vi "cutoff frequency detector.vi"() -> ()   [LabVIEW 2023]
uses:
  ps2000.dll
panel:
  out "Range":dbl
  out "min value":dbl
  out "max value":dbl
  out "Return":string
  in  "error in (no error)":errorcluster
  out "error out":errorcluster
  in  "stop":bool
  out "Waveform Graph":dbl[](graph)
  in  "Trigger Config":T1={"Delay"=0, "Auto_trigger_ms"=0, "Direction"=0, "Source"=5, "Voltage mV"=10} {"Voltage mV" min=0 max=20000 step=50; "Source" items=["Channel A"=0, "Channel B"=1, "Off"=5]; "Direction" items=["Rising", "Falling"]}
  in  "Timebase":cluster{"no_of_samples":i16, "Timebase":i16}
  in  "Apply settings":bool
  in  "Channel A":T2 {"Coupling" items=["DC", "AC"]; "Range" items=["±20 mV"=1, "±50 mV"=2, "±100 mV"=3, "±200 mV"=4, "±500 mV"=5, "±1 V"=6, "±2 V"=7, "±5 V"=8, "±10 V"=9, "±20 V"=10]}
  in  "Channel (1:Channel 1)":u16(ring) items=["", "Channel 1", "Channel 2"]
  in  "DG811 Config":T3
  in  "Waveform Function (0: Sine)":u16(ring) items=["Sine", "Square", "Ramp", "Pulse", "Noise", "DC "]
  in  "Address":refnum<visa-resource-name>
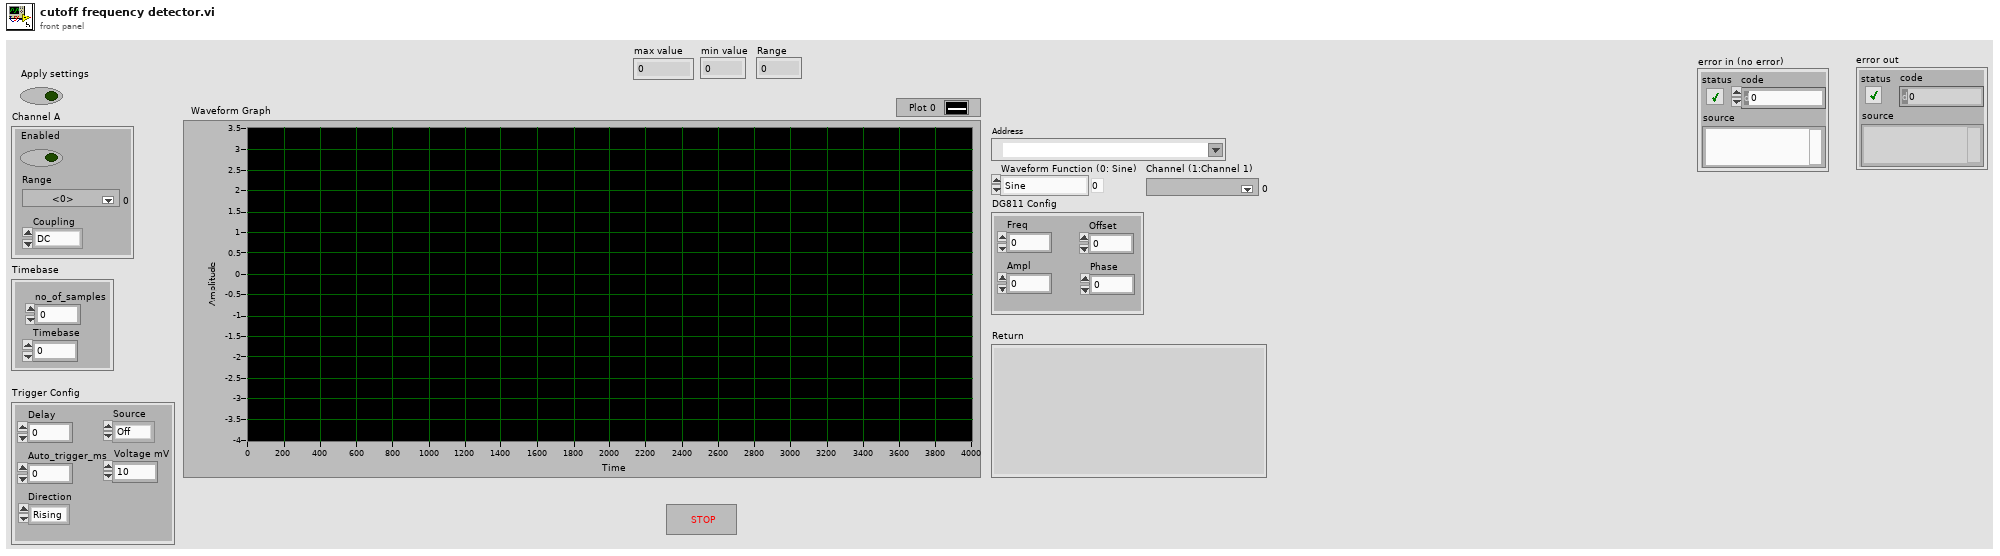
[diagram p1: front panel]
types:
  T1 = cluster{"Delay":i16, "Auto_trigger_ms":i16, "Direction":i16, "Source":i16, "Voltage mV":i16}
  T2 = cluster{"Range":i16, "Enabled":bool, "Coupling":i16}
  T3 = cluster{"Offset ":i8, "Phase ":i8, "Ampl ":i8, "Freq ":i16}
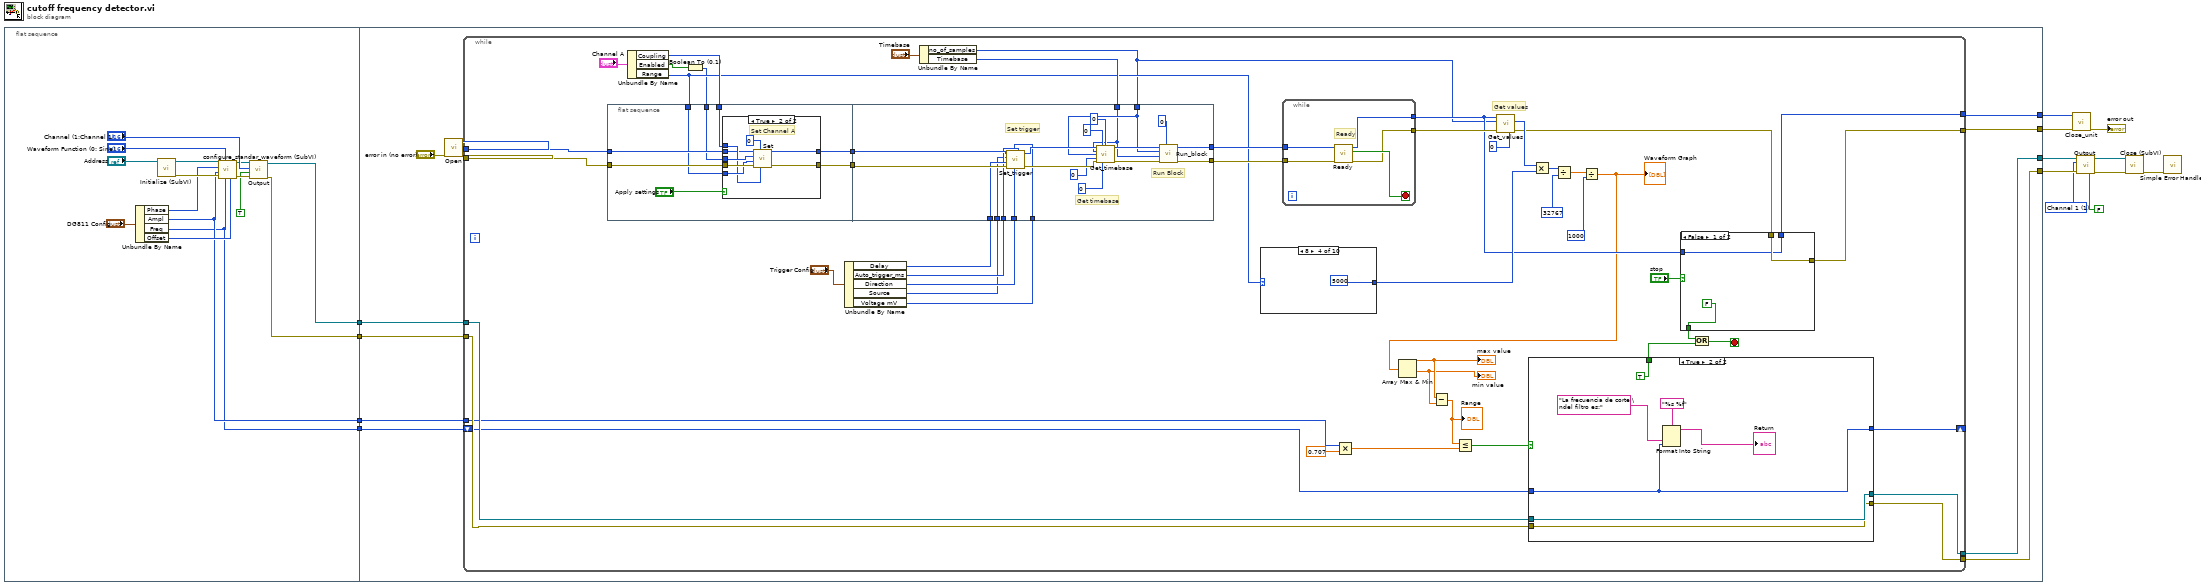
[diagram p0: block diagram]
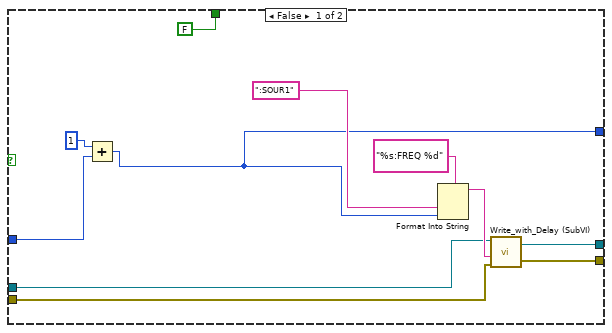
[diagram p2: hidden frame]
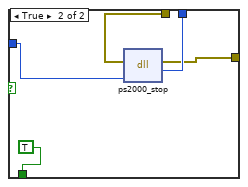
[diagram p3: hidden frame]
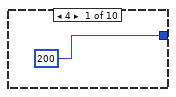
[diagram p5: hidden frame]
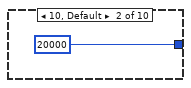
[diagram p6: hidden frame]
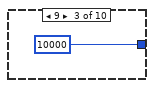
[diagram p7: hidden frame]
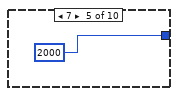
[diagram p8: hidden frame]
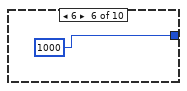
[diagram p9: hidden frame]
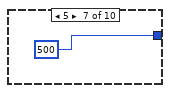
[diagram p10: hidden frame]
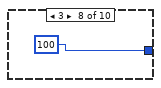
[diagram p11: hidden frame]
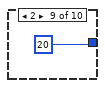
[diagram p12: hidden frame]
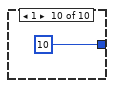
[diagram p13: hidden frame]
diagram:
  w5 = 1 items=["", "Channel 1", "Channel 2"] ("Channel (0: Channel 1)")
  n1 = flat-sequence {
    tunnel: [w22] -> w10
    tunnel: [w21] -> w9
    tunnel: [w16] -> w8
    tunnel: [w15] -> w1
    tunnel: [w37] -> w12
    tunnel: [w36] -> w11
    tunnel: w10 -> [w35]
    tunnel: w9 -> [w34]
    tunnel: [w33] -> w7
    tunnel: [w32] -> w6
    tunnel: w8 -> [w31]
    tunnel: w1 -> [w30]
    frame #0 {
      n2 = Unbundle By Name("DG811 Config") -> ("Phase"=w18:i8, "Ampl"=w16:i8, "Freq"=w15:i16, "Offset"=w17:i8)
      n3 = call "Initialize (SubVI).vi"("VISA Refnum in"="Address") -> ("error out"=w26:errorcluster, "VISA Refnum out"=w25:refnum<visa-resource-name>)  [unwired: 9 in]
      n4 = call "configure_standar_waveform (SubVI).vi"("DC Offset (0 V)"=w17, "Frequency (1000 Hz)"=w15, "Waveform Function (0: Sine) in"="Waveform Function (0: Sine)", "error in (no error)"=w26, "Amplitude (5.0 Vpp)"=w16, "Phase"=w18, "VISA Refnum in"=w25) -> ("error out"=w27:errorcluster, "VISA Refnum out"=w28:refnum<visa-resource-name>)  [unwired: 3 in]
      n5 = call "Output.vi"("error in (no error)"=w27, "Enable Output (T: Enable)"=TRUE, "Channel (0: Channel 1)"="Channel (1:Channel 1)", "VISA Refnum in"=w28) -> ("error out"=w21:errorcluster, "VISA Refnum out"=w22:refnum<visa-resource-name>)  [unwired: 6 in]
    }
    frame #1 {
      n6 = call "Open.vi"("error in (no error)"="error in (no error)") -> ("error out"=w39:errorcluster, "return type"=w38:i16)  [unwired: 9 in]
      n7 = while {
        tunnel: [w78] -> w36
        tunnel: w39 -> [w81]
        tunnel: w38 -> [w82]
        tunnel: [w77] -> w37
        tunnel: w35 -> [w59]
        tunnel: w34 -> [w58]
        tunnel: [w60] -> w33
        tunnel: [w61] -> w32
        tunnel: w31 -> [w46]
        shift-right: [w57] -> _
        shift-left: w30 -> [w56]
        stop <- w54 stop-if-true
        # "Get values"
        n8 = flat-sequence {
          tunnel: w81 -> [w128]
          tunnel: [w127] -> w90
          tunnel: [w126] -> w89
          tunnel: w82 -> [w125]
          tunnel: w73 -> [w124]
          tunnel: w72 -> [w123]
          tunnel: w70 -> [w122]
          tunnel: w90 -> [w151]
          tunnel: w89 -> [w159]
          tunnel: [w158] -> w88
          tunnel: [w148] -> w86
          tunnel: w52 -> [w146]
          tunnel: w75 -> [w145]
          tunnel: w68 -> [w144]
          tunnel: w67 -> [w143]
          tunnel: w66 -> [w142]
          tunnel: w65 -> [w141]
          tunnel: w64 -> [w140]
          frame #0 {
            n9 = case shown="True" "Apply settings" {
              tunnel: w128 -> [w131 w139]
              tunnel: w122 -> [_ w136]
              tunnel: w124 -> [_ w134]
              tunnel: [w130 w132] -> w127
              tunnel: [w131 w138] -> w126
              tunnel: w125 -> [w130 w133]
              tunnel: w123 -> [_ w135]
              frame False {
              }
              frame True {
                # "Set Channel A"
                n10 = call "Set.vi"("DC"=w134, "Channel"=i16 0, "error in (no error)"=w139, "Range"=w135, "enabled"=w136, "Handle"=w133) -> ("error out"=w138:errorcluster, "Return Type"=w132:i16)  [unwired: 4 in]
              }
            }
          }
          frame #1 {
            # "Run Block"
            # "Set trigger"
            # "Get timebase"
            n11 = call "Set_trigger.vi"("Auto_trigger_ms"=w143, "Direction"=w142, "Threshold"=w140, "error in (no error)"=w159, "Delay"=w144, "Source"=w141, "Handle"=w151) -> ("error out"=w157:errorcluster, "return type"=w150:i16)  [unwired: 3 in]
            n12 = call "Get_timebase.vi"("Handle"=w150, "*time_interval"=i16 0, "Oversample"=i16 0, "TimeBase"=w145, "no_of_samples"=w146, "*Max_samples"=i16 0, "error in (no error)"=w157, "*time_units"=i16 0) -> ("return type"=w149:i16, "error out"=w156:errorcluster)  [unwired: 6 in]
            n13 = call "Run_block.vi"("Oversample"=i16 0, "error in (no error)"=w156, "Timebase"=w145, "no_of_samples"=w146, "Handle"=w149) -> ("error out"=w158:errorcluster, "return type"=w148:i16)  [unwired: 5 in]
          }
        }
        n14 = Unbundle By Name("Channel A") -> ("Coupling"=w73:i16, "Enabled"=w71:bool, "Range"=w72:i16)
        n15 = Boolean To (0,1)(Boolean=w71) -> (0, 1=w70:i16)
        n16 = Unbundle By Name("Trigger Config") -> ("Delay"=w68:i16, "Auto_trigger_ms"=w67:i16, "Direction"=w66:i16, "Source"=w65:i16, "Voltage mV"=w64:i16)
        n17 = Unbundle By Name("Timebase") -> ("no_of_samples"=w52:i16, "Timebase"=w75:i16)
        n18 = case shown="8" w72 {
          tunnel: [200 20000 10000 5000 2000 1000 500 100 20 10] -> w85
          frame 4 {
          }
          frame 10, Default {
          }
          frame 9 {
          }
          frame 8 {
          }
          frame 7 {
          }
          frame 6 {
          }
          frame 5 {
          }
          frame 3 {
          }
          frame 2 {
          }
          frame 1 {
          }
        }
        n19 = while {
          tunnel: w88 -> [w120]
          tunnel: [w119] -> w87
          tunnel: w86 -> [w118]
          tunnel: [w117] -> w63
          stop <- w121 stop-if-true
          # "Ready"
          n20 = call "Ready.vi"("error in (no error)"=w120, "Handle"=w118) -> ("error out"=w119:errorcluster, "x != 0?"=w121:bool, "return type"=w117:i16)  [unwired: 7 in]
        }
        n21 = Multiply(x=w46, y=0.707) -> (x*y=w42:dbl)
        n22 = call "Get_values.vi"("*Overflow"=i16 0, "error in (no error)"=w87, "No Of Samples"=w52, "Handle"=w63) -> ("error out"=w79:errorcluster, "*Buffer_a"=w84:i16[])  [unwired: 4 in, 2 out]
        n23 = Multiply(x=w84, y=w85) -> (x*y=w50:i32[])
        n24 = Divide(x=w50, y=32767) -> (x/y=w48:dbl[])
        n25 = Divide(x=w48, y=1000) -> (x/y=w47:dbl[])
        "Waveform Graph" <- w47
        n26 = Array Max & Min(array=w47) -> (max value=w45:dbl, min value=w44:dbl)  [unwired: 2 out]
        "min value" <- w44
        "max value" <- w45
        n27 = Subtract(x=w45, y=w44) -> (x-y=w43:dbl)
        "Range" <- w43
        n28 = Less Or Equal?(x=w43, y=w42) -> (x <= y?=w41:bool)
        n29 = case shown="True" w41 {
          tunnel: [w98 w107] -> w61
          tunnel: [w97 w108] -> w60
          tunnel: w59 -> [w96 w108]
          tunnel: w58 -> [w95 w107]
          tunnel: [w91 w104] -> w57
          tunnel: w56 -> [w92 w104]
          tunnel: [FALSE TRUE] -> w53
          frame False {
            n30 = Add(x=i16 1, y=w92) -> (x+y=w91:i16)
            n31 = Format Into String(format string="%s:FREQ %d", ":SOUR1", w91) -> (resulting string=w99:string)  [unwired: 2 in, 1 out]
            n32 = call "Write_with_Delay (SubVI).vi"("error in (no error)"=w95, "Command"=w99, "VISA Refnum in"=w96) -> ("error out"=w98:errorcluster, "VISA Refnum out"=w97:refnum<visa-resource-name>)  [unwired: 1 in]
          }
          frame True {
            n33 = Format Into String(format string="%s %f", "La frecuencia de corte \ndel filtro es:" ("input 1"), w104) -> (resulting string=→"Return":string)  [unwired: 2 in, 1 out]
          }
        }
        n34 = case shown="False" "stop" {
          tunnel: [FALSE TRUE] -> w55
          tunnel: w79 -> [w110 w115]
          tunnel: [w109 w114] -> w78
          tunnel: [w110 w113] -> w77
          tunnel: w63 -> [w109 w112]
          frame False {
          }
          frame True {
            n35 = dll-call lib="C:/Users/cesar/Desktop/Ps2000 library/ps2000.dll" fn="ps2000_stop"(error in=w115, "handle"=w112) -> (error out=w113:errorcluster, "return type"=w114:i16)  [unwired: 3 in, 1 out]
          }
        }
        n36 = Or(x=w55, y=w53) -> (x .or. y?=w54:bool)
      }
    }
  }
  n37 = call "Close_unit.vi"("error in (no error)"=w12, "Handle"=w11) -> ("error out"=→"error out":errorcluster)  [unwired: 9 in]
  n38 = call "Output.vi"("error in (no error)"=w6, "Enable Output (T: Enable)"=FALSE, "Channel (0: Channel 1)"=w5, "VISA Refnum in"=w7) -> ("error out"=w2:errorcluster, "VISA Refnum out"=w3:refnum<visa-resource-name>)  [unwired: 6 in]
  n39 = call "Close (SubVI).vi"("error in (no error)"=w2, "VISA Refnum in"=w3) -> ("error out"=w14:errorcluster)  [unwired: 9 in]
  n40 = call <vilib>:"Simple Error Handler.vi"("error in (no error)"=w14) -> ()  [unwired: 1 in, 8 out]
